vi "PCF8591.so Path.vi"() -> (1 "PCF8591.so Path":path=path "pcf8591.so")   [LabVIEW 2014, in "QwaveSys Raspberry Pi Library.lvlib"]
uses:
  QwaveSys Raspberry Pi Library.lvlib
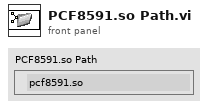
[diagram p1: front panel]
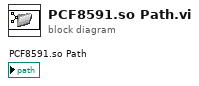
[diagram p0: block diagram]
diagram:
